vi "test.vi"() -> ()   [LabVIEW 2022 SP3, in "SingleStepCODMnV2.lvlib" / "SingleStepCODMnV2.lvclass"]
uses:
  SingleStepCODMnV2.lvclass
panel:
  in  "单步调试":T1={"模式选择"=enum."测试模式", "测试模式"={"进样:"=enum."未选择", "偏心轮: "=0, "注射泵:"=enum."未选择", "量: "=5000, "缺液检测"=FALSE, "外设:"={"排液"=FALSE, "搅拌"=FALSE, "风扇"=FALSE, "废液分离"=FALSE}, "加热:"=FALSE, "摄氏度"=0, "阀配置"=0}, "流程模式"={"功能选择"=enum."注入", "阀口选择"=enum."未选择", "外设"={"排液阀"=FALSE, "搅拌"=FALSE, "冷凝风扇"=FALSE, "废液分离阀"=FALSE, "电磁阀1"=FALSE, "电磁阀2"=FALSE, "电磁阀3"=FALSE, "电磁阀4"=FALSE, "电磁阀5"=FALSE, "电磁阀6"=FALSE, "电磁阀7"=FALSE, "顺时针"=FALSE, "逆时针"=FALSE}, "其他"=enum."未选择", "柱塞泵体积μL"=5000, "摄氏度"=0, "加热:"=FALSE}} {"测试模式"."阀配置" items=["三通阀", "排阀"]}
  in  "模式选择 2":enum16{"测试模式", "流程模式"}(ring)=enum."流程模式"
  out "模式选择":enum16{"测试模式", "流程模式"}(ring)
  out "数组":u16[](array[numeric])
  in  "布尔":bool
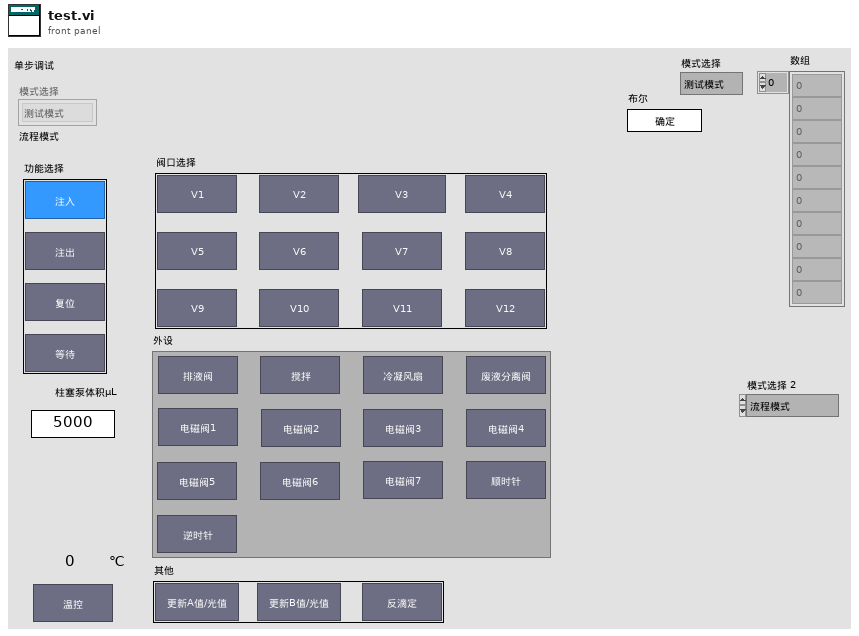
[diagram p1: front panel]
types:
  T1 = cluster{"模式选择":enum16{"测试模式", "流程模式"}, "测试模式":cluster{"进样:":enum32{"未选择", "水样", "纯水", "标液", "零点", "加标回收", "跨度"}, "偏心轮: ":u16, "注射泵:":enum32{"未选择", "纯水-进", "纯水-排", "硫酸-进", "硫酸-排", "复位", "高锰酸钾-进", "高锰酸钾-排", "草酸钠-进", "草酸钠-排", "氢氧化钠-进", "氢氧化钠-排", "反滴定"}, "量: ":u16, "缺液检测":bool, "外设:":cluster{"排液":bool, "搅拌":bool, "风扇":bool, "废液分离":bool}, "加热:":bool, "摄氏度":u16, "阀配置":u8}, "流程模式":cluster{"功能选择":enum32{"等待", "复位", "注入", "注出"}, "阀口选择":enum32{"未选择", "V1", "V2", "V3", "V4", "V5", "V6", "V7", "V8", "V9", "V10", "V11", "V12"}, "外设":cluster{"排液阀":bool, "搅拌":bool, "冷凝风扇":bool, "废液分离阀":bool, "电磁阀1":bool, "电磁阀2":bool, "电磁阀3":bool, "电磁阀4":bool, "电磁阀5":bool, "电磁阀6":bool, "电磁阀7":bool, "顺时针":bool, "逆时针":bool}, "其他":enum32{"未选择", "更新A值", "更新B值", "反滴定"}, "柱塞泵体积μL":u16, "摄氏度":u16, "加热:":bool}}
  T2 = cluster{"监测参数":u8, "模式选择 2":enum16{"测试模式", "流程模式"}}
  T3 = cluster{"数组":u16[], "模式选择":enum16{"测试模式", "流程模式"}}
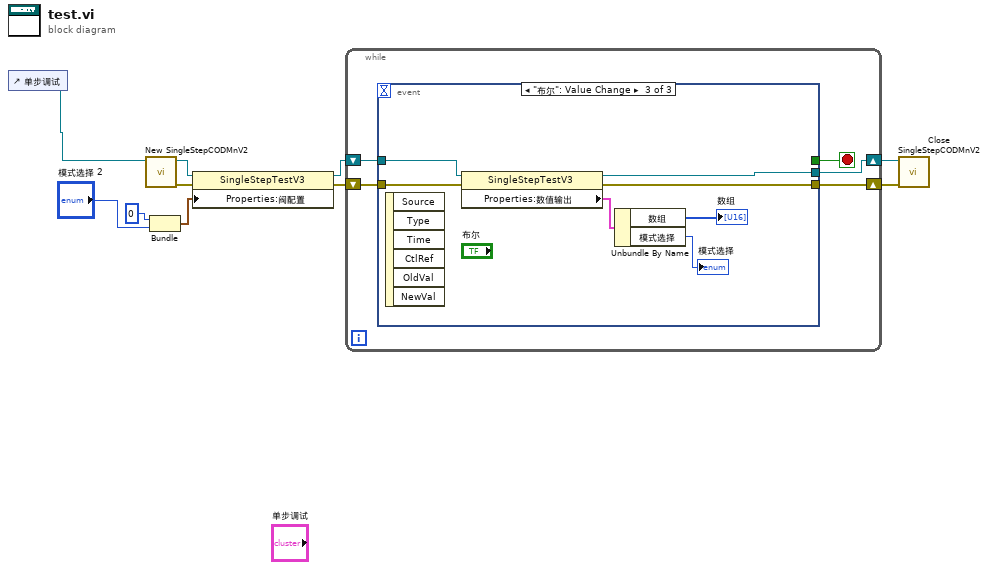
[diagram p0: block diagram]
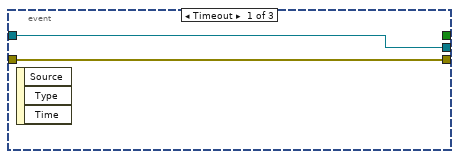
[diagram p2: hidden frame]
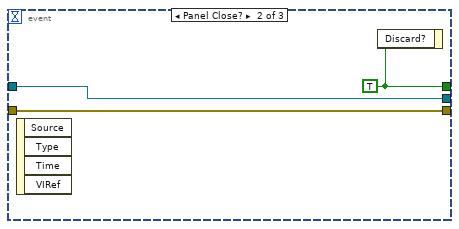
[diagram p3: hidden frame]
diagram:
  n1 = control-ref of="单步调试"() -> (w1:refnum<vi>)
  n2 = call "New SingleStepCODMnV2.vi"("Reference"=w1) -> ("error out"=w8:errorcluster, "SingleStepTestV3 out"=w5:refnum<class "SingleStepCODMnV2.lvclass">)  [unwired: 9 in]
  n3 = Bundle("监测参数"=u8 0, "模式选择 2"="模式选择 2") -> (w2:T2)  [unwired: 1 in]
  n4 = property class="SingleStepTestV3"(reference=w5, error in=w8, "Properties:阀配置"=w2) -> (reference out=w7:refnum<class "SingleStepCODMnV2.lvclass">, error out=w6:errorcluster)
  n5 = while {
    shift-right: [w12] -> w10
    shift-left: w7 -> [w15]
    shift-right: [w11] -> w9
    shift-left: w6 -> [w14]
    stop <- w13 stop-if-true
    n6 = event shown="[2] \"布尔\": Value Change" {
      selector: _ -> [_ _ _]
      dyn-events: _ -> [_ _ _]
      timeout: _ -> [_ _ _]
      tunnel: w15 -> [w17 w19 w27]
      tunnel: w14 -> [w16 w18 w24]
      tunnel: [_ w20 _] -> w13
      tunnel: [w17 w19 w26] -> w12
      tunnel: [w16 w18 w25] -> w11
      event Timeout {
        n7 = event-data() -> ()  [unwired: 1 in, 3 out]
      }
      event Panel Close? {
        w20 = TRUE
        n8 = event-data() -> ()  [unwired: 1 in, 4 out]
        n9 = event-data("Discard?"=w20) -> ()  [unwired: 1 in, 1 out]
      }
      event "布尔": Value Change {
        n10 = event-data() -> ()  [unwired: 1 in, 6 out]
        n11 = property class="SingleStepTestV3"(reference=w27, error in=w24) -> (reference out=w26:refnum<class "SingleStepCODMnV2.lvclass">, error out=w25:errorcluster, "Properties:数值输出"=w23:T3)
        n12 = Unbundle By Name(w23) -> ("数组"=→"数组":u16[], "模式选择"=→"模式选择":enum16{"测试模式", "流程模式"})
      }
    }
  }
  n13 = call "Close SingleStepCODMnV2.vi"("error in (no error)"=w9, "SingleStepTestV3 in"=w10) -> ()  [unwired: 9 in, 1 out]
